vi "disconnectCommandSubscribe.vi"(8 "error in (no error)":errorcluster, 11 "MiddlewareSALThisComponent in":refnum<class "MiddlewareSALThisComponent.lvclass">) -> (0 "error out":errorcluster, 3 "MiddlewareSALThisComponent out":refnum<class "MiddlewareSALThisComponent.lvclass">)   [LabVIEW 2016, in "MiddlewareSALThisComponent.lvclass"]
uses:
  MiddlewareSALThisComponent.lvclass
  ProgrammaticInitialization/ProgrammaticInitialization.lvclass
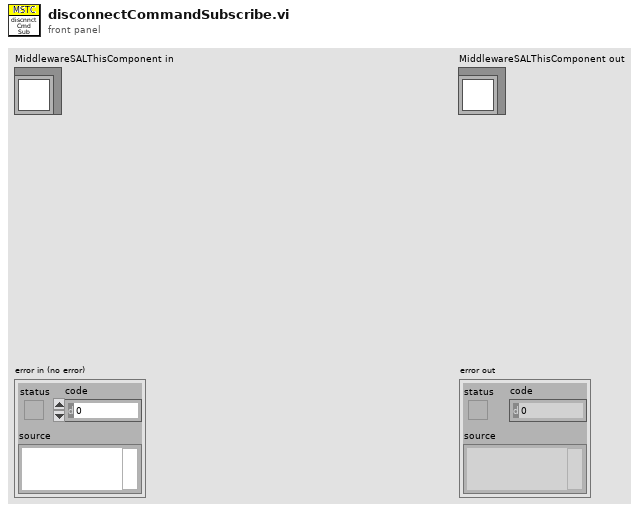
[diagram p1: front panel]
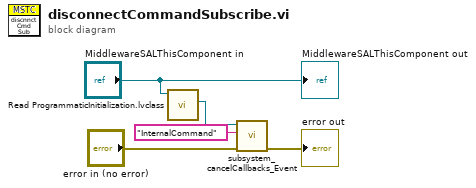
[diagram p0: block diagram]
diagram:
  n1 = call-dynamic "Read ProgrammaticInitialization.lvclass.vi"("MiddlewareSALThisComponent in"="MiddlewareSALThisComponent in") -> ("ProgrammaticInitialization.lvclass"=w2:refnum<class "ProgrammaticInitialization.lvclass">)  [unwired: 8 in, 2 out]
  n2 = call "subsystem_cancelCallbacks_Event.vi"("error in (no error)"="error in (no error)", "topic"="InternalCommand", "ProgrammaticInitialization in"=w2) -> ("error out"=→"error out":errorcluster)  [unwired: 7 in, 1 out]
  "MiddlewareSALThisComponent out" <- "MiddlewareSALThisComponent in"
